vi "parse_AccelStamped.vi"(4 "error in":errorcluster, 7 "msg in":string) -> (0 "error out":errorcluster, 1 "Vector":T1, 2 "Header":T2, 3 "msg out":string)   [LabVIEW 2016]
doc: "Parses a message into an acceleration stamped"
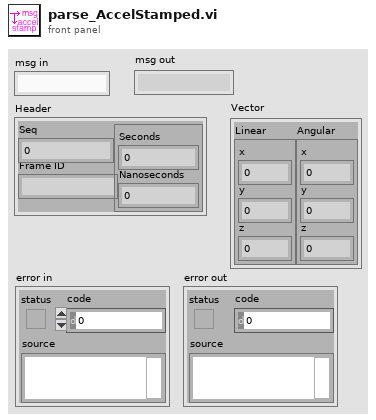
[diagram p1: front panel]
types:
  T1 = cluster{"Linear":cluster{"x":dbl, "y":dbl, "z":dbl}, "Angular":cluster{"x":dbl, "y":dbl, "z":dbl}}
  T2 = cluster{"Seq":u32, "Frame ID":string, "Timestamp":cluster{"Seconds":i32, "Nanoseconds":i32}}
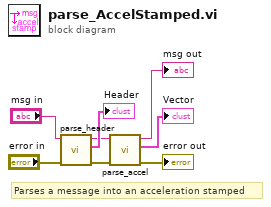
[diagram p0: block diagram]
diagram:
  # "Parses a message into an acceleration stamped"
  n1 = call "parse_header.vi"("error in"="error in", "msg in"="msg in") -> ("error out"=w4:errorcluster, "Header"=→"Header":T2, "msg out"=w5:string)  [unwired: 3 in]
  n2 = call "parse_accel.vi"("error in"=w4, "msg in"=w5) -> ("error out"=→"error out":errorcluster, "Accel"=→"Vector":T1, "msg out"=→"msg out":string)  [unwired: 3 in]
